vi "探头数据读取.vi"(11 "编号":string) -> ()   [LabVIEW 2016, in "斯坦道多参数.lvlib"]
panel:
  out "运行状态":u16(ring) items=["空闲", "水样测试", "标样核查"]
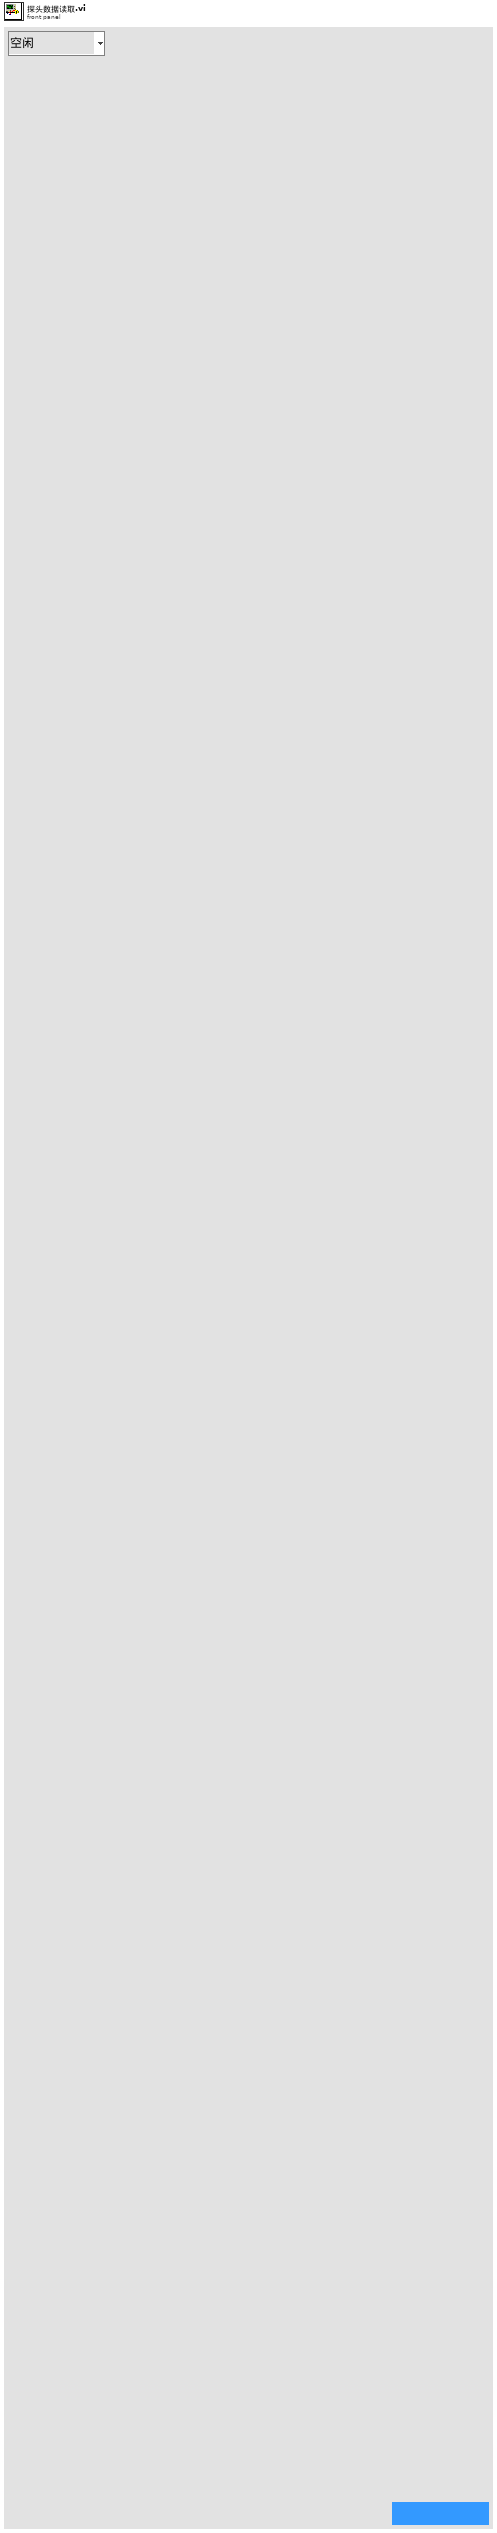
[diagram p1: front panel]
types:
  T1 = enum16{"pH", "DO", "Cond", "Turb", "ORP", "叶绿素a", "藻密度"}
  T2 = cluster{"温度测量值":sgl, "测量值":sgl, "温度偏移修正值":sgl, "信号值":sgl}
  T3 = cluster{"温度测量值":sgl, "DO%":sgl, "DOmg/L":sgl, "温度偏移修正值":sgl}
  T4 = cluster{"CH":u16, "监测值":dbl, "温度偏移修正值":sgl, "信号值":sgl}
  T5 = cluster{"pH探头选择":u16, "DO探头选择":u16, "电导率探头选择":u16, "浊度探头选择":u16, "叶绿素a探头选择":u16, "蓝绿藻探头选择":u16, "orp探头选择":u16}
  T6 = cluster{"电极状态标志":u16, "电极型号标志":u16, "酸碱度测量值":sgl, "温度测量值":sgl, "酸碱度信号值":sgl, "温度信号值":sgl, "酸碱度偏移修正值":sgl, "温度偏移修正值":sgl, "手动温度补偿值":sgl, "酸碱度电极零点":sgl, "酸碱度电极斜率":sgl, "第1点标准值记录":sgl, "第1点信号值记录":sgl, "第1点温度值记录":sgl, "第2点标准值记录":sgl, "第2点信号值记录":sgl, "第2点温度值记录":sgl, "命令滤波设定":u16, "温度模式":enum16{"ATC", "MTC"}, "生产批次":u16, "电极序号":u16, "串口地址":u16, "串口波特率":enum16{"9600", "19200", "115200"}, "串口校验位":enum16{"NONE", "ODD", "EVEN"}, "串口停止位":enum16{"1bit", "2bit"}, "第一点标准值":sgl, "第二点标准值":sgl}
  T7 = cluster{"报警码":u16, "pH数值":sgl, "0X0003_NC":sgl, "温度数据":sgl, "pH原始信号 mv":sgl, "0X0009_NC":string, "产品名称":string, "序列号":string, "硬件版本":string, "软件版本":string, "通讯地址":u16, "波特率":u16, "设备类型":u16, "0X0026_NC":string, "第一点原始数据":sgl, "第一点校准数据":sgl, "第二点原始数据":sgl, "第二点校准数据":sgl, "探头校准命令":u16, "温度校准参数":sgl, "温度校准命令":u16}
  T8 = cluster{"电极状态标志":u16, "电极型号标志":u16, "电导率测量值":sgl, "温度测量值":sgl, "电导率信号值":sgl, "温度信号值":sgl, "温度补偿系数":sgl, "电导率偏移修正值":sgl, "温度偏移修正值":sgl, "手动温度补偿值":sgl, "电导率电极零点":sgl, "电导率电极斜率":sgl, "命令滤波设定":u16, "温度模式":enum16{"ATC", "MTC"}, "生产批次":u16, "电极序号":u16, "串口地址":u16, "串口波特率":enum16{"9600", "19200", "115200"}, "串口校验位":enum16{"NONE", "ODD", "EVEN"}, "串口停止位":enum16{"1bit", "2bit"}, "第一点标准值":sgl, "第二点标准值":sgl}
  T9 = cluster{"报警码":u16, "电导率数据（uS/cm）":sgl, "0x0003 NC":sgl, "温度数据":sgl, "电导率原始信号电阻":sgl, "当前量程":u16, "温度补偿系数":sgl, "0X0009_NC":string, "产品名称":string, "序列号":string, "硬件版本":string, "软件版本":string, "通讯地址":u16, "波特率":u16, "设备类型":u16, "0X0026_NC":string, "第一点原始数据":sgl, "第一点校准数据":sgl, "0X0035_NC":sgl, "0X0037_NC":sgl, "探头校准命令":u16, "温度校准参数":sgl, "温度校准命令":u16}
  T10 = cluster{"电极状态标志":u16, "电极型号标志":u16, "溶解氧测量值":sgl, "温度测量值":sgl, "溶解氧饱和度值":sgl, "盐度补偿值":sgl, "大气压补偿值":sgl, "溶解氧偏移修正值":sgl, "温度偏移修正值":sgl, "手动温度补偿值":sgl, "溶解氧电极零点":sgl, "溶解氧电极斜率":sgl, "第1点标准值记录":sgl, "第1点信号值记录":sgl, "第1点温度值记录":sgl, "第2点标准值记录":sgl, "第2点信号值记录":sgl, "第2点温度值记录":sgl, "命令滤波设定":u16, "温度模式":enum16{"ATC", "MTC"}, "生产批次":u16, "电极序号":u16, "串口地址":u16, "串口波特率":enum16{"9600", "19200", "115200"}, "串口校验位":enum16{"NONE", "ODD", "EVEN"}, "串口停止位":enum16{"1bit", "2bit"}, "第一点标准值":sgl, "第二点标准值":sgl}
  T11 = cluster{"报警码":u16, "溶解氧数值（mg/L）":sgl, "溶解氧数据（%）":sgl, "温度数据":sgl, "溶解氧原始信号 nA":sgl, "大气压力":sgl, "盐度":sgl, "0X0009_NC":string, "产品名称":string, "序列号":string, "硬件版本":string, "软件版本":string, "通讯地址":u16, "波特率":u16, "设备类型":u16, "0X0026_NC":string, "第一点原始数据":sgl, "0X0033 NC":sgl, "第二点原始数据":sgl, "0X0037 NC":sgl, "探头校准命令":u16, "温度校准参数":sgl, "温度校准命令":u16}
  T12 = cluster{"电极状态标志":u16, "电极型号标志":u16, "浊度测量值":sgl, "温度测量值":sgl, "浊度信号值":sgl, "浊度偏移修正值":sgl, "温度偏移修正值":sgl, "手动温度补偿值":sgl, "浊度电极零点":sgl, "浊度电极斜率":sgl, "第1点标准值记录":sgl, "第1点信号值记录":sgl, "第1点温度值记录":sgl, "第2点标准值记录":sgl, "第2点信号值记录":sgl, "第2点温度值记录":sgl, "命令滤波设定":u16, "温度模式":enum16{"ATC", "MTC"}, "生产批次":u16, "电极序号":u16, "串口地址":u16, "串口波特率":enum16{"9600", "19200", "115200"}, "串口校验位":enum16{"NONE", "ODD", "EVEN"}, "串口停止位":enum16{"1bit", "2bit"}, "第一点标准值":sgl, "第二点标准值":sgl, "第三点标准值":sgl}
  T13 = cluster{"报警码":u16, "浊度数值 NTU":sgl, "温度数据":sgl, "原始光强数值":u16, "量程":u16, "平均次数":u16, "清扫模式":u16, "清扫次数":u16, "清扫间隔分钟":u16, "0X000B_NC":string, "产品名称":string, "序列号":string, "硬件版本":string, "软件版本":string, "通讯地址":u16, "波特率":u16, "设备类型":u16, "0X0026_NC":string, "校准量程":u16, "第一点原始光强":u16, "第一点校准数据":sgl, "第二点原始光强":u16, "第二点校准数据":sgl, "第三点原始光强":u16, "第三点校准数据":sgl, "探头校准命令":u16, "温度校准参数":sgl, "温度校准命令":u16}
  T14 = cluster{"电极状态标志":u16, "电极型号标志":u16, "测量值":sgl, "温度测量值":sgl, "信号值":sgl, "温度信号值":sgl, "000AH_NC":sgl, "偏移修正值":sgl, "温度偏移修正值":sgl, "手动温度补偿值":sgl, "命令滤波设定":u16, "温度模式":enum16{"ATC", "MTC"}, "生产批次":u16, "传感器序号":u16, "串口地址":u16, "串口波特率":enum16{"9600", "19200", "115200"}, "串口校验位":enum16{"NONE", "ODD", "EVEN"}, "串口停止位":enum16{"1bit", "2bit"}}
  T15 = cluster{"报警码":u16, "叶绿素a":sgl, "温度数据":sgl, "原始光强数值":u16, "量程":u16, "平均次数":u16, "清扫模式":u16, "清扫次数":u16, "清扫间隔分钟":u16, "0X000B_NC":string, "产品名称":string, "序列号":string, "硬件版本":string, "软件版本":string, "通讯地址":u16, "波特率":u16, "设备类型":u16, "0X0026_NC":string, "校准量程":u16, "第一点原始光强":u16, "第一点校准数据":sgl, "第二点原始光强":u16, "第二点校准数据":sgl, "第三点原始光强":u16, "第三点校准数据":sgl, "探头校准命令":u16, "温度校准参数":sgl, "温度校准命令":u16}
  T16 = cluster{"报警码":u16, "蓝绿藻":sgl, "温度数据":sgl, "原始光强数值":u16, "0X0006_NC":u16, "平均次数":u16, "清扫模式":u16, "清扫次数":u16, "清扫间隔分钟":u16, "0X000B_NC":string, "产品名称":string, "序列号":string, "硬件版本":string, "软件版本":string, "通讯地址":u16, "波特率":u16, "设备类型":u16, "0X0026_NC":string, "0X0030_NC":u16, "第一点原始光强":u16, "第一点校准数据":sgl, "第二点原始光强":u16, "第二点校准数据":sgl, "第三点原始光强":u16, "第三点校准数据":sgl, "探头校准命令":u16, "温度校准参数":sgl, "温度校准命令":u16}
  T17 = enum16{"pH", "DO", "Cond", "Turb", "ORP", "叶绿素a", "藻密度"}[]
  T18 = cluster{"ph":bool, "DO":bool, "Cond":bool, "Turb":bool, "叶绿素a":bool, "藻密度":bool, "ORP":bool}
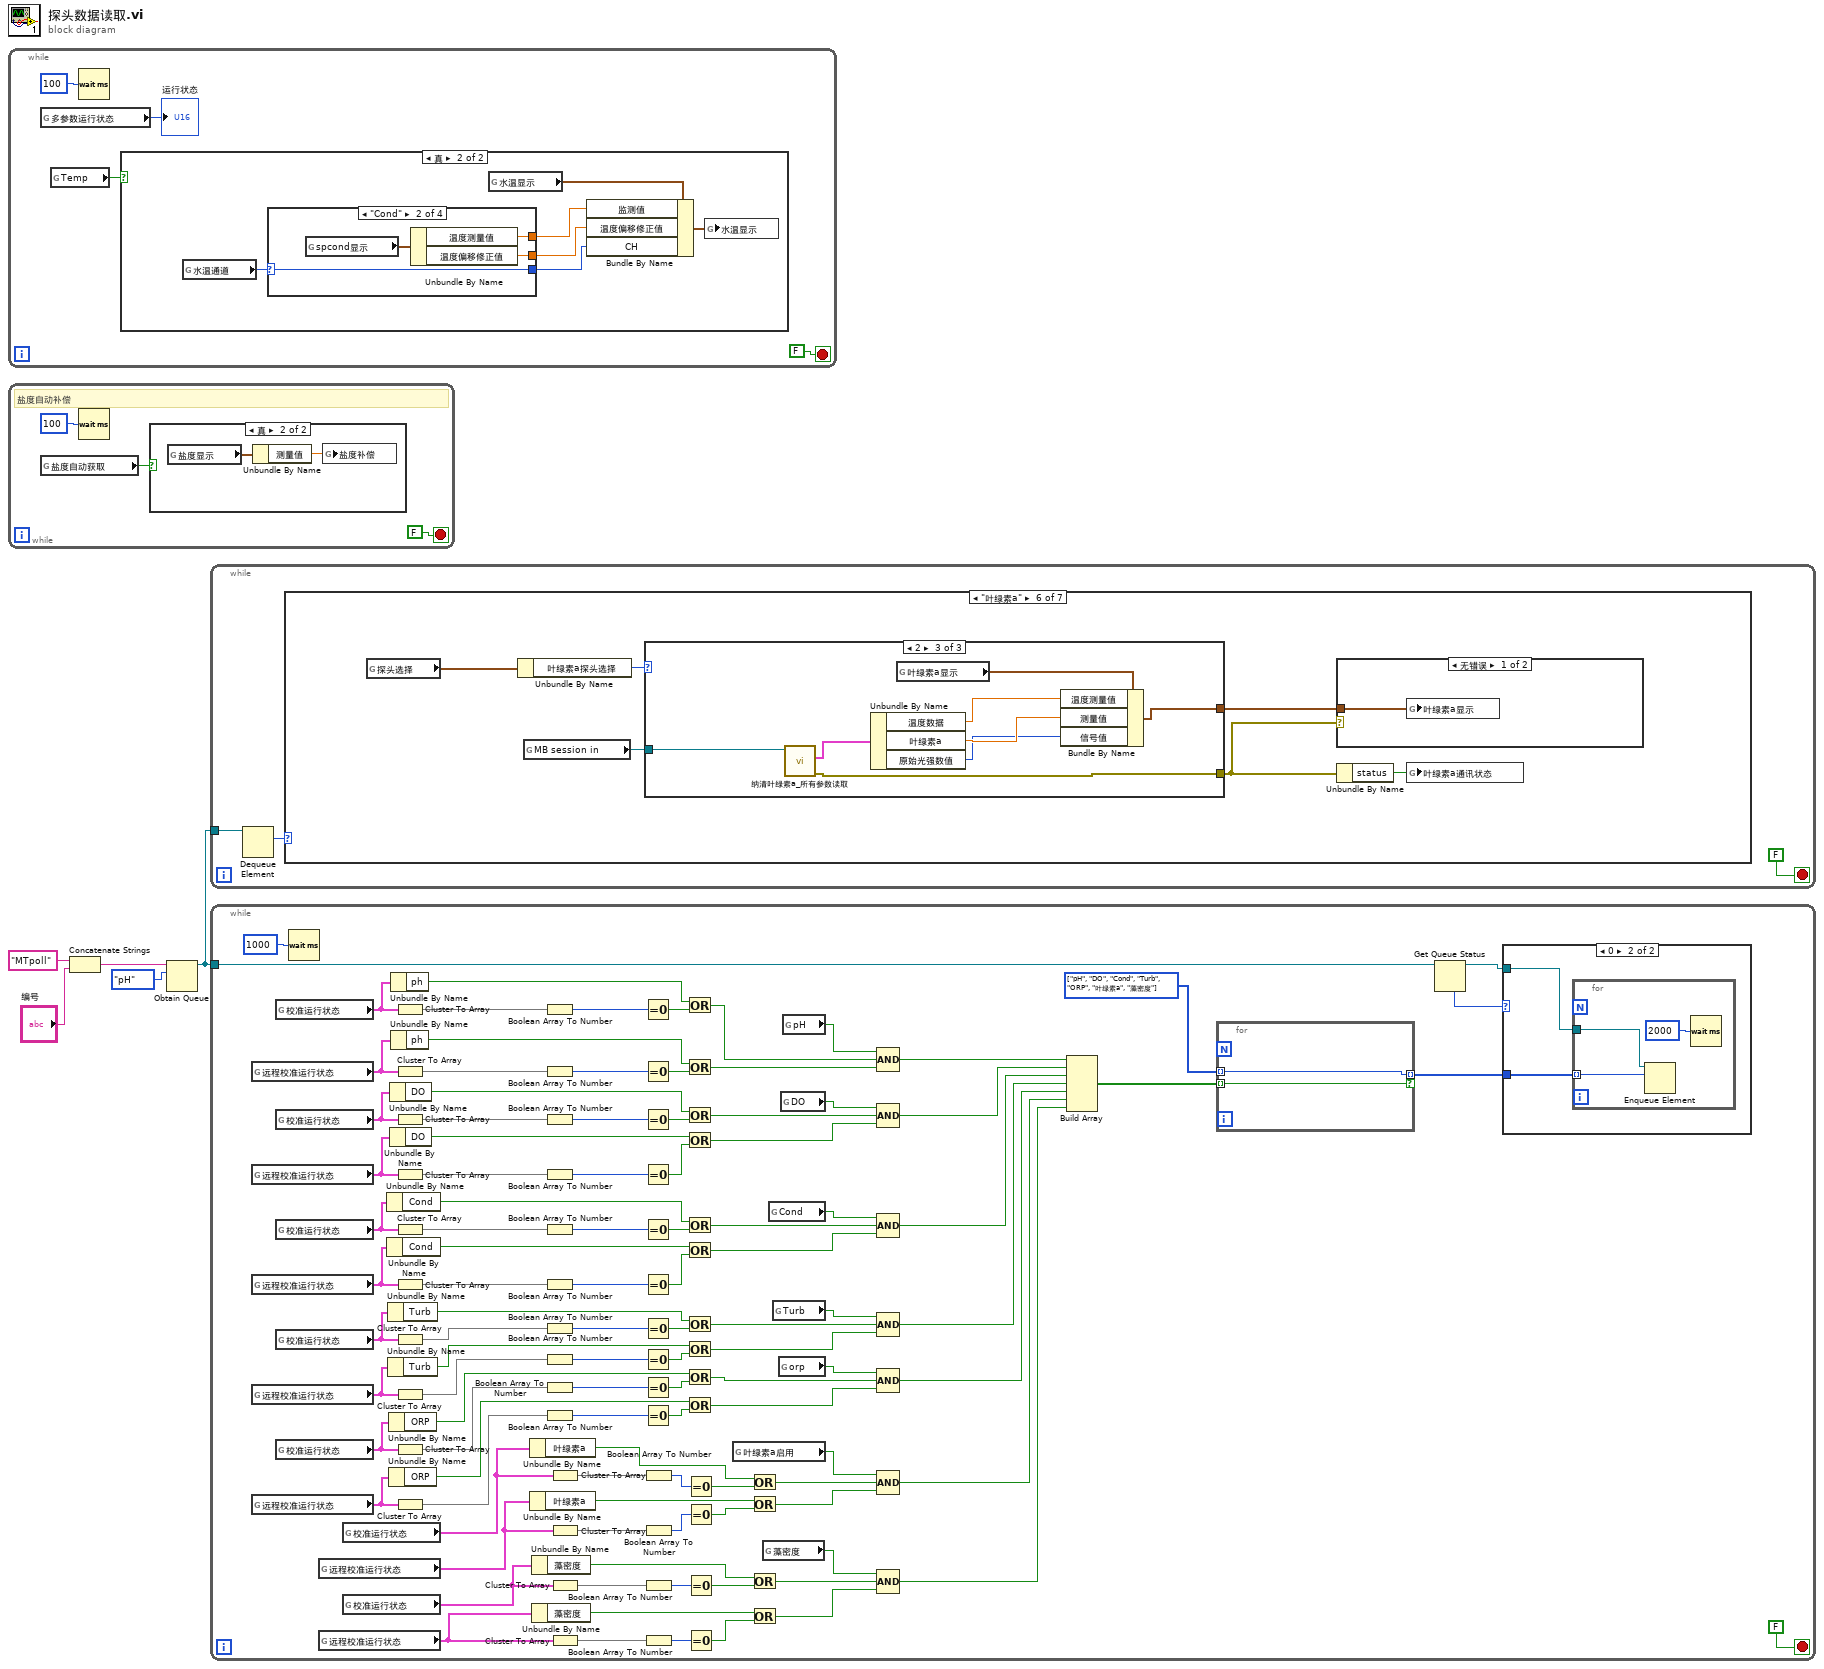
[diagram p0: block diagram]
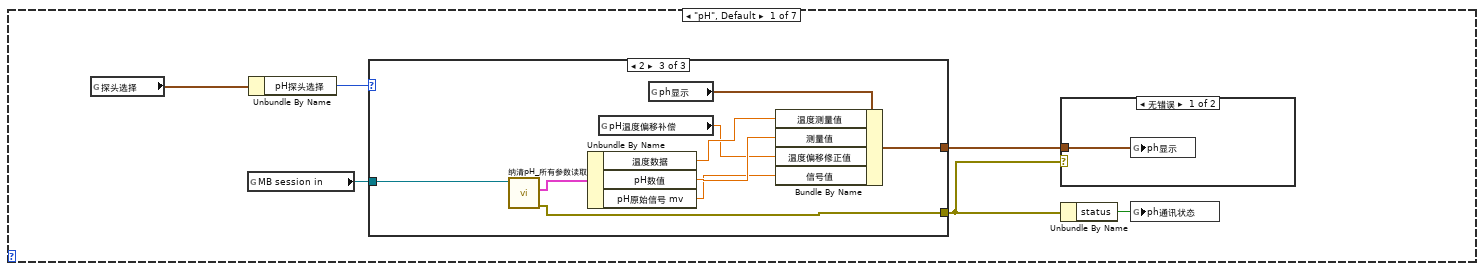
[diagram p3: hidden frame]
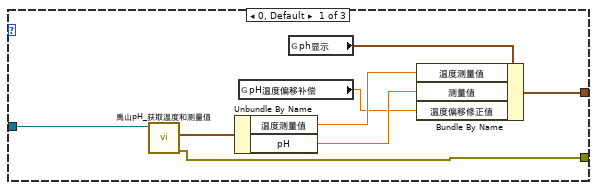
[diagram p4: hidden frame]
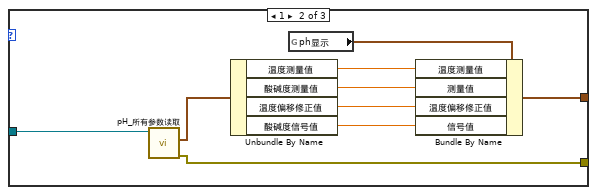
[diagram p5: hidden frame]
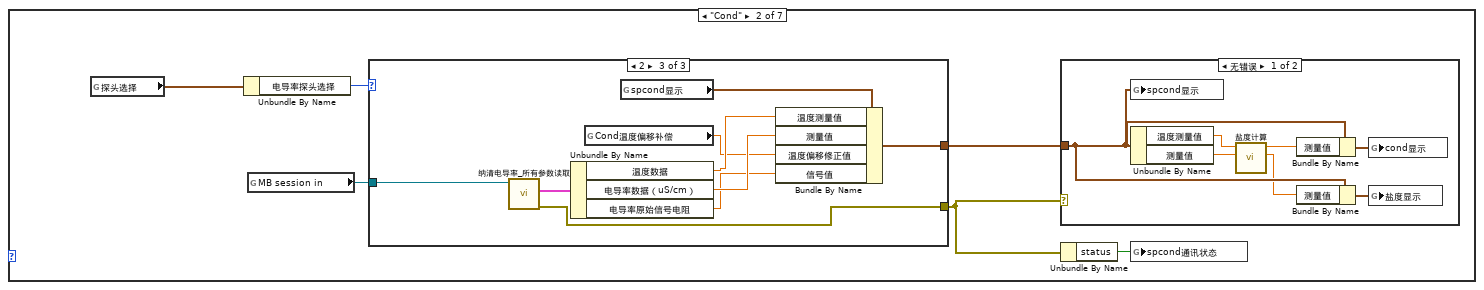
[diagram p7: hidden frame]
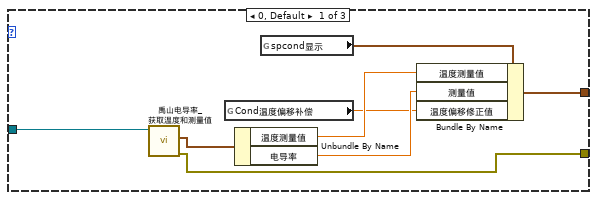
[diagram p8: hidden frame]
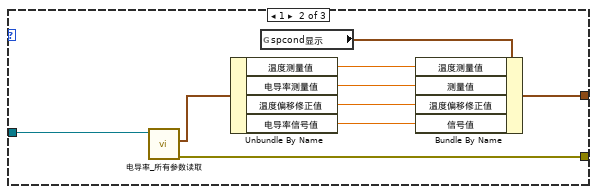
[diagram p9: hidden frame]
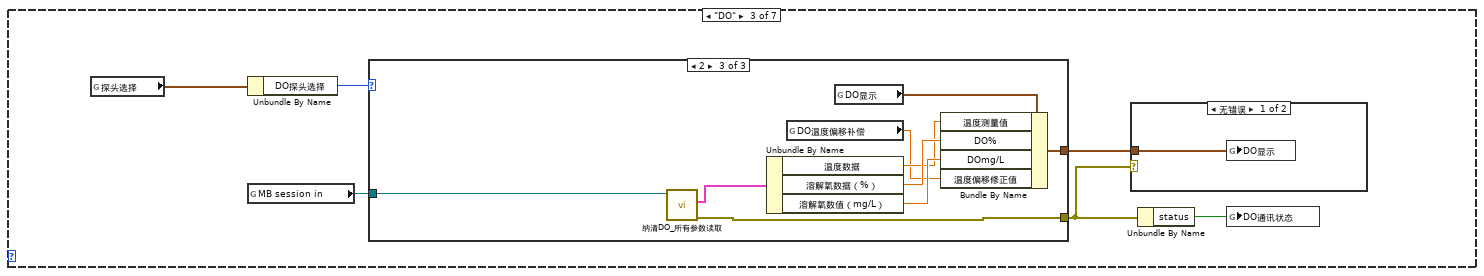
[diagram p11: hidden frame]
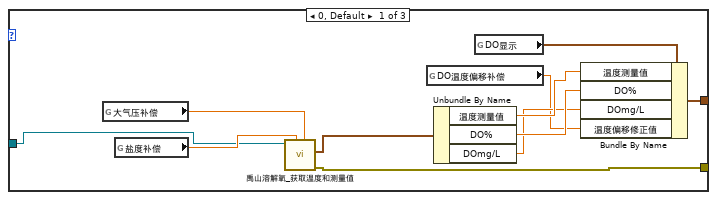
[diagram p12: hidden frame]
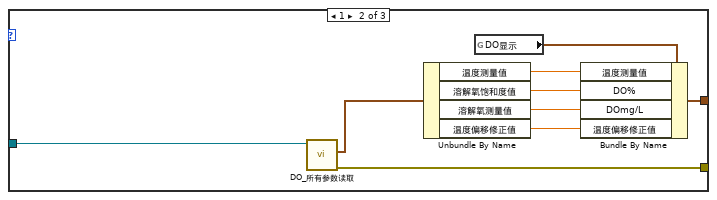
[diagram p13: hidden frame]
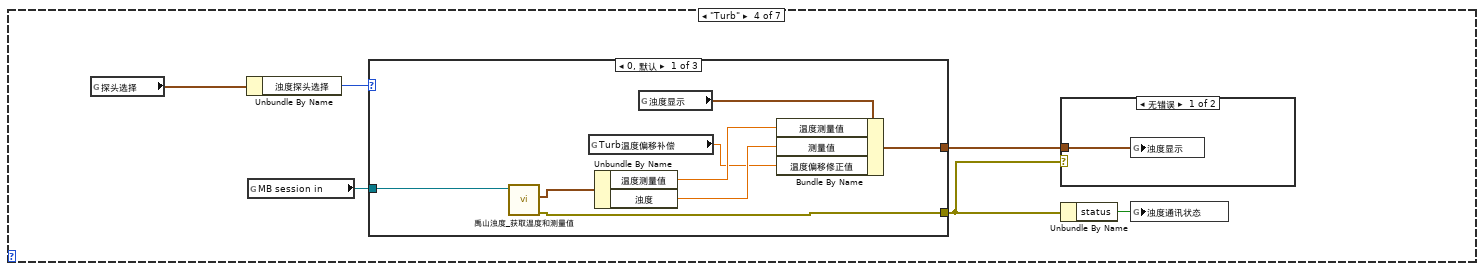
[diagram p15: hidden frame]
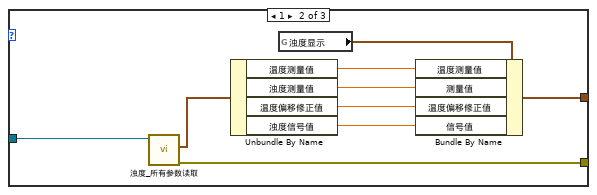
[diagram p16: hidden frame]
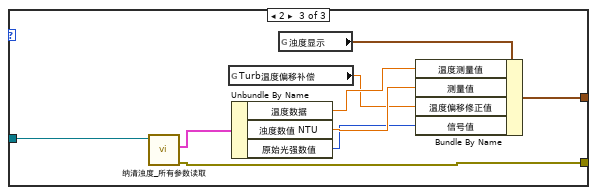
[diagram p17: hidden frame]
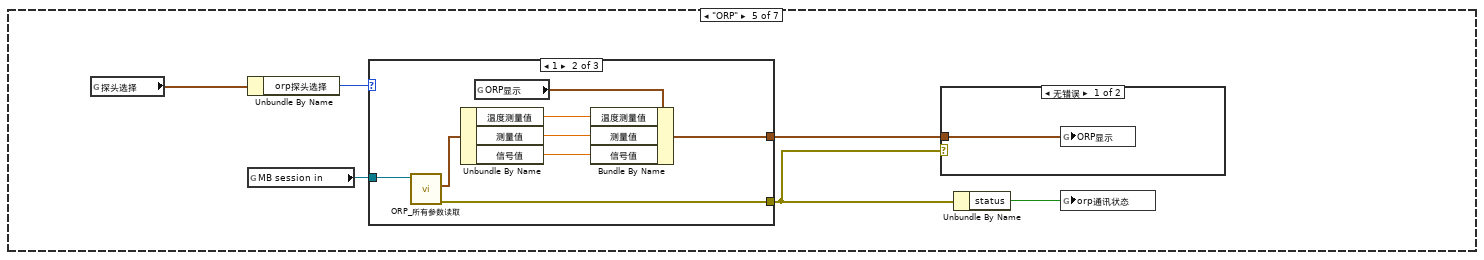
[diagram p19: hidden frame]
diagram:
  n1 = while {
    stop <- FALSE stop-if-true
    n2 = global read "多参数全局变量.vi" "多参数运行状态"() -> (→"运行状态":u16)
    n3 = global read "断电保存变量.vi" "Temp"() -> (w7:bool)
    n4 = Wait (ms)(milliseconds to wait=u32 100 ("等待时间（毫秒）")) -> ()  [unwired: 1 out]
    n5 = case shown="真" w7 {
      frame False {
      }
      frame True {
        n6 = global read "断电保存变量.vi" "水温通道"() -> (w15:enum16{"pH", "Cond", "DO", "Turb"})
        n7 = case shown="\"Cond\"" w15 {
          selector: w15 -> [w19 w23 w27 w31]
          tunnel: [w19 w23 w27 w31] -> w14
          tunnel: [w17 w20 w24 w28] -> w13
          tunnel: [w18 w21 w25 w29] -> w12
          frame "pH", Default {
            n8 = global read "多参数全局变量.vi" "ph显示"() -> (w16:T2)
            n9 = Unbundle By Name(w16) -> ("温度测量值"=w18:sgl, "温度偏移修正值"=w17:sgl)
          }
          frame "Cond" {
            n10 = global read "多参数全局变量.vi" "spcond显示"() -> (w22:T2)
            n11 = Unbundle By Name(w22) -> ("温度测量值"=w21:sgl, "温度偏移修正值"=w20:sgl)
          }
          frame "DO" {
            n12 = global read "多参数全局变量.vi" "DO显示"() -> (w26:T3)
            n13 = Unbundle By Name(w26) -> ("温度测量值"=w25:sgl, "温度偏移修正值"=w24:sgl)
          }
          frame "Turb" {
            n14 = global read "多参数全局变量.vi" "浊度显示"() -> (w30:T2)
            n15 = Unbundle By Name(w30) -> ("温度测量值"=w29:sgl, "温度偏移修正值"=w28:sgl)
          }
        }
        n16 = global read "多参数全局变量.vi" "水温显示"() -> (w10:T4)
        n17 = Bundle By Name(cluster=w10, "监测值"=w12, "温度偏移修正值"=w13, "CH"=w14) -> (w11:T4)
        n18 = global write "多参数全局变量.vi" "水温显示"(w11) -> ()
      }
    }
  }
  n19 = while {
    stop <- FALSE stop-if-true
    # "盐度自动补偿"
    n20 = global read "断电保存变量.vi" "盐度自动获取"() -> (w33:bool)
    n21 = Wait (ms)(milliseconds to wait=u32 100 ("等待时间（毫秒）")) -> ()  [unwired: 1 out]
    n22 = case shown="真" w33 {
      frame False {
      }
      frame True {
        n23 = global read "多参数全局变量.vi" "盐度显示"() -> (w36:T2)
        n24 = Unbundle By Name(w36) -> ("测量值"=w35:sgl)
        n25 = global write "断电保存变量.vi" "盐度补偿"(w35) -> ()
      }
    }
  }
  n26 = Concatenate Strings("MTpoll" ("名称（未命名）"), "编号") -> (w3:string)
  n27 = Obtain Queue(name (unnamed)=w3, element data type=T1."pH" ("枚举")) -> (queue out=w1:refnum<queue>)  [unwired: 3 in, 2 out]
  n28 = while {
    tunnel: w1 -> [w39]
    stop <- FALSE stop-if-true
    n29 = Dequeue Element(queue=w39) -> (element=w38:T1)  [unwired: 2 in, 3 out]
    n30 = case shown="\"叶绿素a\"" w38 {
      frame "pH", Default {
        n31 = global read "断电保存变量.vi" "探头选择"() -> (w45:T5)
        n32 = global read "多参数全局变量.vi" "MB session in"() -> (w43:refnum<class "MB_Master.lvclass">)
        n33 = Unbundle By Name(w45) -> ("pH探头选择"=w44:u16)
        n34 = case shown="2" w44 {
          tunnel: w43 -> [w53 w62 w69]
          tunnel: [w52 w61 w67] -> w41
          tunnel: [w50 w58 w70] -> w42
          frame 0, Default {
            n35 = call "禹山pH_获取温度和测量值.vi"("MB session in"=w53) -> ("error out"=w52:errorcluster, "输出值"=w49:cluster{"温度测量值":sgl, "ORP":sgl, "pH":sgl})  [unwired: 8 in, 1 out]
            n36 = Unbundle By Name(w49) -> ("温度测量值"=w48:sgl, "pH"=w47:sgl)
            n37 = global read "断电保存变量.vi" "pH温度偏移补偿"() -> (w46:dbl)
            n38 = global read "多参数全局变量.vi" "ph显示"() -> (w51:T2)
            n39 = Bundle By Name(cluster=w51, "温度测量值"=w48, "测量值"=w47, "温度偏移修正值"=w46) -> (w50:T2)
          }
          frame 1 {
            n40 = call "pH_所有参数读取.vi"("MB session in"=w62) -> ("error out"=w61:errorcluster, "输出值"=w60:T6)  [unwired: 8 in, 1 out]
            n41 = Unbundle By Name(w60) -> ("温度测量值"=w55:sgl, "酸碱度测量值"=w56:sgl, "温度偏移修正值"=w57:sgl, "酸碱度信号值"=w54:sgl)
            n42 = global read "多参数全局变量.vi" "ph显示"() -> (w59:T2)
            n43 = Bundle By Name(cluster=w59, "温度测量值"=w55, "测量值"=w56, "温度偏移修正值"=w57, "信号值"=w54) -> (w58:T2)
          }
          frame 2 {
            n44 = call "纳清pH_所有参数读取.vi"("MB session in"=w69) -> ("error out"=w67:errorcluster, "输出值"=w68:T7)  [unwired: 8 in, 1 out]
            n45 = Unbundle By Name(w68) -> ("温度数据"=w66:sgl, "pH数值"=w65:sgl, "pH原始信号 mv"=w63:sgl)
            n46 = global read "断电保存变量.vi" "pH温度偏移补偿"() -> (w64:dbl)
            n47 = global read "多参数全局变量.vi" "ph显示"() -> (w71:T2)
            n48 = Bundle By Name(cluster=w71, "温度测量值"=w66, "测量值"=w65, "温度偏移修正值"=w64, "信号值"=w63) -> (w70:T2)
          }
        }
        n49 = case shown="无错误" w41 {
          tunnel: w42 -> [w72 _]
          frame No Error {
            n50 = global write "多参数全局变量.vi" "ph显示"(w72) -> ()
          }
          frame Error {
          }
        }
        n51 = Unbundle By Name(w41) -> ("status"=w40:bool)
        n52 = global write "多参数全局变量.vi" "ph通讯状态"(w40) -> ()
      }
      frame "Cond" {
        n53 = global read "断电保存变量.vi" "探头选择"() -> (w78:T5)
        n54 = Unbundle By Name(w78) -> ("电导率探头选择"=w77:u16)
        n55 = global read "多参数全局变量.vi" "MB session in"() -> (w75:refnum<class "MB_Master.lvclass">)
        n56 = case shown="2" w77 {
          tunnel: w75 -> [w86 w95 w100]
          tunnel: [w80 w93 w103] -> w76
          tunnel: [w85 w92 w98] -> w74
          frame 0, Default {
            n57 = call "禹山电导率_获取温度和测量值.vi"("MB session in"=w86) -> ("error out"=w85:errorcluster, "输出值"=w83:cluster{"温度测量值":sgl, "电导率":sgl, "错误标志":u16})  [unwired: 8 in, 1 out]
            n58 = global read "断电保存变量.vi" "Cond温度偏移补偿"() -> (w79:dbl)
            n59 = Unbundle By Name(w83) -> ("温度测量值"=w82:sgl, "电导率"=w81:sgl)
            n60 = global read "多参数全局变量.vi" "spcond显示"() -> (w84:T2)
            n61 = Bundle By Name(cluster=w84, "温度测量值"=w82, "测量值"=w81, "温度偏移修正值"=w79) -> (w80:T2)
          }
          frame 1 {
            n62 = call "电导率_所有参数读取.vi"("MB session in"=w95) -> ("error out"=w92:errorcluster, "输出值"=w91:T8)  [unwired: 8 in, 1 out]
            n63 = Unbundle By Name(w91) -> ("温度测量值"=w90:sgl, "电导率测量值"=w89:sgl, "温度偏移修正值"=w88:sgl, "电导率信号值"=w87:sgl)
            n64 = global read "多参数全局变量.vi" "spcond显示"() -> (w94:T2)
            n65 = Bundle By Name(cluster=w94, "温度测量值"=w90, "测量值"=w89, "温度偏移修正值"=w88, "信号值"=w87) -> (w93:T2)
          }
          frame 2 {
            n66 = call "纳清电导率_所有参数读取.vi"("MB session in"=w100) -> ("error out"=w98:errorcluster, "输出值"=w99:T9)  [unwired: 8 in, 1 out]
            n67 = Unbundle By Name(w99) -> ("温度数据"=w102:sgl, "电导率数据（uS/cm）"=w101:sgl, "电导率原始信号电阻"=w96:sgl)
            n68 = global read "断电保存变量.vi" "Cond温度偏移补偿"() -> (w97:dbl)
            n69 = global read "多参数全局变量.vi" "spcond显示"() -> (w104:T2)
            n70 = Bundle By Name(cluster=w104, "温度测量值"=w102, "测量值"=w101, "温度偏移修正值"=w97, "信号值"=w96) -> (w103:T2)
          }
        }
        n71 = case shown="无错误" w74 {
          tunnel: w76 -> [w106 _]
          frame No Error {
            n72 = global write "多参数全局变量.vi" "spcond显示"(w106) -> ()
            n73 = Unbundle By Name(w106) -> ("温度测量值"=w111:sgl, "测量值"=w110:sgl)
            n74 = call "盐度计算.vi"("spCond"=w110, "Temp"=w111) -> ("saltresult"=w105:dbl, "cond"=w109:dbl)  [unwired: 8 in]
            n75 = Bundle By Name(cluster=w106, "测量值"=w109) -> (w108:T2)
            n76 = Bundle By Name(cluster=w106, "测量值"=w105) -> (w107:T2)
            n77 = global write "多参数全局变量.vi" "cond显示"(w108) -> ()
            n78 = global write "多参数全局变量.vi" "盐度显示"(w107) -> ()
          }
          frame Error {
          }
        }
        n79 = Unbundle By Name(w74) -> ("status"=w73:bool)
        n80 = global write "多参数全局变量.vi" "spcond通讯状态"(w73) -> ()
      }
      frame "DO" {
        n81 = global read "断电保存变量.vi" "探头选择"() -> (w117:T5)
        n82 = Unbundle By Name(w117) -> ("DO探头选择"=w116:u16)
        n83 = global read "多参数全局变量.vi" "MB session in"() -> (w114:refnum<class "MB_Master.lvclass">)
        n84 = case shown="2" w116 {
          tunnel: w114 -> [w126 w137 w141]
          tunnel: [w124 w135 w145] -> w115
          tunnel: [w120 w130 w139] -> w113
          frame 0, Default {
            n85 = global read "断电保存变量.vi" "大气压补偿"() -> (w127:dbl)
            n86 = global read "断电保存变量.vi" "盐度补偿"() -> (w128:dbl)
            n87 = call "禹山溶解氧_获取温度和测量值.vi"("大气压补偿"=w127, "盐度补偿"=w128, "MB session in"=w126) -> ("error out"=w120:errorcluster, "输出值"=w118:cluster{"温度测量值":sgl, "DO%":sgl, "DOmg/L":sgl})  [unwired: 6 in, 1 out]
            n88 = global read "断电保存变量.vi" "DO温度偏移补偿"() -> (w119:dbl)
            n89 = Unbundle By Name(w118) -> ("温度测量值"=w123:sgl, "DO%"=w122:sgl, "DOmg/L"=w121:sgl)
            n90 = global read "多参数全局变量.vi" "DO显示"() -> (w125:T3)
            n91 = Bundle By Name(cluster=w125, "温度测量值"=w123, "DO%"=w122, "DOmg/L"=w121, "温度偏移修正值"=w119) -> (w124:T3)
          }
          frame 1 {
            n92 = call "DO_所有参数读取.vi"("MB session in"=w137) -> ("error out"=w130:errorcluster, "输出值"=w134:T10)  [unwired: 8 in, 1 out]
            n93 = Unbundle By Name(w134) -> ("温度测量值"=w131:sgl, "溶解氧饱和度值"=w132:sgl, "溶解氧测量值"=w133:sgl, "温度偏移修正值"=w129:sgl)
            n94 = global read "多参数全局变量.vi" "DO显示"() -> (w136:T3)
            n95 = Bundle By Name(cluster=w136, "温度测量值"=w131, "DO%"=w132, "DOmg/L"=w133, "温度偏移修正值"=w129) -> (w135:T3)
          }
          frame 2 {
            n96 = call "纳清DO_所有参数读取.vi"("MB session in"=w141) -> ("error out"=w139:errorcluster, "输出值"=w140:T11)  [unwired: 8 in, 1 out]
            n97 = Unbundle By Name(w140) -> ("温度数据"=w142:sgl, "溶解氧数据（%）"=w143:sgl, "溶解氧数值（mg/L）"=w144:sgl)
            n98 = global read "断电保存变量.vi" "DO温度偏移补偿"() -> (w138:dbl)
            n99 = global read "多参数全局变量.vi" "DO显示"() -> (w146:T3)
            n100 = Bundle By Name(cluster=w146, "温度测量值"=w142, "DO%"=w143, "DOmg/L"=w144, "温度偏移修正值"=w138) -> (w145:T3)
          }
        }
        n101 = case shown="无错误" w113 {
          tunnel: w115 -> [w147 _]
          frame No Error {
            n102 = global write "多参数全局变量.vi" "DO显示"(w147) -> ()
          }
          frame Error {
          }
        }
        n103 = Unbundle By Name(w113) -> ("status"=w112:bool)
        n104 = global write "多参数全局变量.vi" "DO通讯状态"(w112) -> ()
      }
      frame "Turb" {
        n105 = global read "断电保存变量.vi" "探头选择"() -> (w153:T5)
        n106 = Unbundle By Name(w153) -> ("浊度探头选择"=w152:u16)
        n107 = global read "多参数全局变量.vi" "MB session in"() -> (w150:refnum<class "MB_Master.lvclass">)
        n108 = case shown="0, 默认" w152 {
          tunnel: w150 -> [w161 w170 w175]
          tunnel: [w159 w165 w176] -> w151
          tunnel: [w158 w164 w174] -> w149
          frame 0, Default {
            n109 = call "禹山浊度_获取温度和测量值.vi"("MB session in"=w161) -> ("error out"=w158:errorcluster, "输出值"=w157:cluster{"温度测量值":sgl, "浊度":sgl})  [unwired: 8 in, 1 out]
            n110 = global read "断电保存变量.vi" "Turb温度偏移补偿"() -> (w154:dbl)
            n111 = Unbundle By Name(w157) -> ("温度测量值"=w156:sgl, "浊度"=w155:sgl)
            n112 = global read "多参数全局变量.vi" "浊度显示"() -> (w160:T2)
            n113 = Bundle By Name(cluster=w160, "温度测量值"=w156, "测量值"=w155, "温度偏移修正值"=w154) -> (w159:T2)
          }
          frame 1 {
            n114 = call "浊度_所有参数读取.vi"("MB session in"=w170) -> ("error out"=w164:errorcluster, "输出值"=w169:T12)  [unwired: 8 in, 1 out]
            n115 = Unbundle By Name(w169) -> ("温度测量值"=w167:sgl, "浊度测量值"=w166:sgl, "温度偏移修正值"=w163:sgl, "浊度信号值"=w162:sgl)
            n116 = global read "多参数全局变量.vi" "浊度显示"() -> (w168:T2)
            n117 = Bundle By Name(cluster=w168, "温度测量值"=w167, "测量值"=w166, "温度偏移修正值"=w163, "信号值"=w162) -> (w165:T2)
          }
          frame 2 {
            n118 = call "纳清浊度_所有参数读取.vi"("MB session in"=w175) -> ("error out"=w174:errorcluster, "输出值"=w173:T13)  [unwired: 8 in, 1 out]
            n119 = global read "断电保存变量.vi" "Turb温度偏移补偿"() -> (w172:dbl)
            n120 = Unbundle By Name(w173) -> ("温度数据"=w178:sgl, "浊度数值 NTU"=w177:sgl, "原始光强数值"=w171:u16)
            n121 = global read "多参数全局变量.vi" "浊度显示"() -> (w179:T2)
            n122 = Bundle By Name(cluster=w179, "温度测量值"=w178, "测量值"=w177, "温度偏移修正值"=w172, "信号值"=w171) -> (w176:T2)
          }
        }
        n123 = case shown="无错误" w149 {
          tunnel: w151 -> [w180 _]
          frame No Error {
            n124 = global write "多参数全局变量.vi" "浊度显示"(w180) -> ()
          }
          frame Error {
          }
        }
        n125 = Unbundle By Name(w149) -> ("status"=w148:bool)
        n126 = global write "多参数全局变量.vi" "浊度通讯状态"(w148) -> ()
      }
      frame "ORP" {
        n127 = global read "断电保存变量.vi" "探头选择"() -> (w185:T5)
        n128 = Unbundle By Name(w185) -> ("orp探头选择"=w184:u16)
        n129 = global read "多参数全局变量.vi" "MB session in"() -> (w183:refnum<class "MB_Master.lvclass">)
        n130 = case shown="1" w184 {
          tunnel: [_ w189 _] -> w182
          tunnel: w183 -> [_ w194 _]
          tunnel: [_ w187 _] -> w186
          frame 0, Default {
          }
          frame 1 {
            n131 = call "ORP_所有参数读取.vi"("MB session in"=w194) -> ("error out"=w189:errorcluster, "输出值"=w191:T14)  [unwired: 8 in, 1 out]
            n132 = Unbundle By Name(w191) -> ("温度测量值"=w192:sgl, "测量值"=w193:sgl, "信号值"=w188:sgl)
            n133 = global read "多参数全局变量.vi" "ORP显示"() -> (w190:T2)
            n134 = Bundle By Name(cluster=w190, "温度测量值"=w192, "测量值"=w193, "信号值"=w188) -> (w187:T2)
          }
          frame 2 {
          }
        }
        n135 = case shown="无错误" w182 {
          tunnel: w186 -> [w195 _]
          frame No Error {
            n136 = global write "多参数全局变量.vi" "ORP显示"(w195) -> ()
          }
          frame Error {
          }
        }
        n137 = Unbundle By Name(w182) -> ("status"=w181:bool)
        n138 = global write "多参数全局变量.vi" "orp通讯状态"(w181) -> ()
      }
      frame "叶绿素a" {
        n139 = global read "断电保存变量.vi" "探头选择"() -> (w200:T5)
        n140 = Unbundle By Name(w200) -> ("叶绿素a探头选择"=w199:u16)
        n141 = global read "多参数全局变量.vi" "MB session in"() -> (w198:refnum<class "MB_Master.lvclass">)
        n142 = case shown="2" w199 {
          tunnel: [w208 _ w214] -> w197
          tunnel: w198 -> [w207 _ w216]
          tunnel: [w205 _ w213] -> w201
          frame 0, Default {
            n143 = call "叶绿素a_获取温度和叶绿素值.vi"("MB session in"=w207) -> ("error out"=w208:errorcluster, "输出值"=w204:cluster{"温度测量值":sgl, "叶绿素测量值":sgl, "错误标志":u16})  [unwired: 8 in, 1 out]
            n144 = Unbundle By Name(w204) -> ("温度测量值"=w202:sgl, "叶绿素测量值"=w203:sgl)
            n145 = global read "多参数全局变量.vi" "叶绿素a显示"() -> (w206:T2)
            n146 = Bundle By Name(cluster=w206, "温度测量值"=w202, "测量值"=w203) -> (w205:T2)
          }
          frame 1 {
          }
          frame 2 {
            n147 = call "纳清叶绿素a_所有参数读取.vi"("MB session in"=w216) -> ("error out"=w214:errorcluster, "输出值"=w212:T15)  [unwired: 8 in, 1 out]
            n148 = Unbundle By Name(w212) -> ("温度数据"=w210:sgl, "叶绿素a"=w211:sgl, "原始光强数值"=w209:u16)
            n149 = global read "多参数全局变量.vi" "叶绿素a显示"() -> (w215:T2)
            n150 = Bundle By Name(cluster=w215, "温度测量值"=w210, "测量值"=w211, "信号值"=w209) -> (w213:T2)
          }
        }
        n151 = case shown="无错误" w197 {
          tunnel: w201 -> [w217 _]
          frame No Error {
            n152 = global write "多参数全局变量.vi" "叶绿素a显示"(w217) -> ()
          }
          frame Error {
          }
        }
        n153 = Unbundle By Name(w197) -> ("status"=w196:bool)
        n154 = global write "多参数全局变量.vi" "叶绿素a通讯状态"(w196) -> ()
      }
      frame "藻密度" {
        n155 = global read "断电保存变量.vi" "探头选择"() -> (w222:T5)
        n156 = Unbundle By Name(w222) -> ("蓝绿藻探头选择"=w221:u16)
        n157 = global read "多参数全局变量.vi" "MB session in"() -> (w220:refnum<class "MB_Master.lvclass">)
        n158 = case shown="2" w221 {
          tunnel: [_ _ w229] -> w219
          tunnel: w220 -> [_ _ w231]
          tunnel: [_ _ w228] -> w223
          frame 0, Default {
          }
          frame 1 {
          }
          frame 2 {
            n159 = call "纳清蓝绿藻_所有参数读取.vi"("MB session in"=w231) -> ("error out"=w229:errorcluster, "输出值"=w227:T16)  [unwired: 8 in, 1 out]
            n160 = Unbundle By Name(w227) -> ("温度数据"=w226:sgl, "蓝绿藻"=w225:sgl, "原始光强数值"=w224:u16)
            n161 = global read "多参数全局变量.vi" "藻密度显示"() -> (w230:T2)
            n162 = Bundle By Name(cluster=w230, "温度测量值"=w226, "测量值"=w225, "信号值"=w224) -> (w228:T2)
          }
        }
        n163 = case shown="无错误" w219 {
          tunnel: w223 -> [w232 _]
          frame No Error {
            n164 = global write "多参数全局变量.vi" "藻密度显示"(w232) -> ()
          }
          frame Error {
          }
        }
        n165 = Unbundle By Name(w219) -> ("status"=w218:bool)
        n166 = global write "多参数全局变量.vi" "藻密度通讯状态"(w218) -> ()
      }
    }
  }
  n167 = while {
    tunnel: w1 -> [w338]
    stop <- FALSE stop-if-true
    w237 = T17 [enum."pH", enum."DO", enum."Cond", enum."Turb", enum."ORP", enum."叶绿素a", enum."藻密度"] items=["pH", "DO", "Cond", "Turb", "ORP", "叶绿素a", "藻密度"]
    n168 = global read "多参数全局变量.vi" "远程校准运行状态"() -> (w335:T18)
    n169 = global read "多参数全局变量.vi" "远程校准运行状态"() -> (w309:T18)
    n170 = global read "多参数全局变量.vi" "远程校准运行状态"() -> (w312:T18)
    n171 = global read "多参数全局变量.vi" "远程校准运行状态"() -> (w296:T18)
    n172 = global read "多参数全局变量.vi" "远程校准运行状态"() -> (w283:T18)
    n173 = global read "多参数全局变量.vi" "校准运行状态"() -> (w324:T18)
    n174 = global read "多参数全局变量.vi" "校准运行状态"() -> (w298:T18)
    n175 = global read "多参数全局变量.vi" "校准运行状态"() -> (w323:T18)
    n176 = global read "多参数全局变量.vi" "校准运行状态"() -> (w285:T18)
    n177 = global read "多参数全局变量.vi" "校准运行状态"() -> (w272:T18)
    n178 = Wait (ms)(milliseconds to wait=u32 1000 ("等待时间（毫秒）")) -> ()  [unwired: 1 out]
    n179 = global read "多参数全局变量.vi" "远程校准运行状态"() -> (w260:T18)
    n180 = global read "多参数全局变量.vi" "远程校准运行状态"() -> (w257:T18)
    n181 = global read "多参数全局变量.vi" "校准运行状态"() -> (w271:T18)
    n182 = global read "多参数全局变量.vi" "校准运行状态"() -> (w246:T18)
    n183 = Unbundle By Name(w323) -> ("Cond"=w321:bool)
    n184 = Unbundle By Name(w312) -> ("Cond"=w313:bool)
    n185 = Unbundle By Name(w285) -> ("Turb"=w287:bool)
    n186 = Unbundle By Name(w296) -> ("Turb"=w295:bool)
    n187 = Unbundle By Name(w272) -> ("ORP"=w274:bool)
    n188 = Unbundle By Name(w283) -> ("ORP"=w282:bool)
    n189 = Unbundle By Name(w298) -> ("DO"=w300:bool)
    n190 = Unbundle By Name(w309) -> ("DO"=w308:bool)
    n191 = Unbundle By Name(w324) -> ("ph"=w326:bool)
    n192 = Unbundle By Name(w335) -> ("ph"=w334:bool)
    n193 = Cluster To Array(cluster=w324) -> (array=w329:bool[])
    n194 = Cluster To Array(cluster=w335) -> (array=w331:bool[])
    n195 = Cluster To Array(cluster=w298) -> (array=w303:bool[])
    n196 = Cluster To Array(cluster=w309) -> (array=w305:bool[])
    n197 = Cluster To Array(cluster=w323) -> (array=w318:bool[])
    n198 = Cluster To Array(cluster=w312) -> (array=w316:bool[])
    n199 = Cluster To Array(cluster=w285) -> (array=w290:bool[])
    n200 = Cluster To Array(cluster=w296) -> (array=w292:bool[])
    n201 = Cluster To Array(cluster=w272) -> (array=w277:bool[])
    n202 = Cluster To Array(cluster=w283) -> (array=w279:bool[])
    n203 = Unbundle By Name(w271) -> ("叶绿素a"=w269:bool)
    n204 = Unbundle By Name(w260) -> ("叶绿素a"=w261:bool)
    n205 = Unbundle By Name(w246) -> ("藻密度"=w248:bool)
    n206 = Unbundle By Name(w257) -> ("藻密度"=w256:bool)
    n207 = Boolean Array To Number(Boolean array=w329) -> (number=w328:u32)
    n208 = Boolean Array To Number(Boolean array=w331) -> (number=w332:u32)
    n209 = Boolean Array To Number(Boolean array=w303) -> (number=w302:u32)
    n210 = Boolean Array To Number(Boolean array=w305) -> (number=w306:u32)
    n211 = Boolean Array To Number(Boolean array=w318) -> (number=w319:u32)
    n212 = Boolean Array To Number(Boolean array=w316) -> (number=w315:u32)
    n213 = Boolean Array To Number(Boolean array=w290) -> (number=w289:u32)
    n214 = Boolean Array To Number(Boolean array=w292) -> (number=w293:u32)
    n215 = Boolean Array To Number(Boolean array=w277) -> (number=w276:u32)
    n216 = Boolean Array To Number(Boolean array=w279) -> (number=w280:u32)
    n217 = Cluster To Array(cluster=w271) -> (array=w266:bool[])
    n218 = Cluster To Array(cluster=w260) -> (array=w264:bool[])
    n219 = Cluster To Array(cluster=w246) -> (array=w251:bool[])
    n220 = Cluster To Array(cluster=w257) -> (array=w253:bool[])
    n221 = Equal To 0?(x=w328) -> (x = 0?=w327:bool)
    n222 = Equal To 0?(x=w332) -> (x = 0?=w333:bool)
    n223 = Equal To 0?(x=w302) -> (x = 0?=w301:bool)
    n224 = Equal To 0?(x=w306) -> (x = 0?=w307:bool)
    n225 = Equal To 0?(x=w319) -> (x = 0?=w320:bool)
    n226 = Equal To 0?(x=w315) -> (x = 0?=w314:bool)
    n227 = Equal To 0?(x=w289) -> (x = 0?=w288:bool)
    n228 = Equal To 0?(x=w293) -> (x = 0?=w294:bool)
    n229 = Equal To 0?(x=w276) -> (x = 0?=w275:bool)
    n230 = Equal To 0?(x=w280) -> (x = 0?=w281:bool)
    n231 = Boolean Array To Number(Boolean array=w266) -> (number=w267:u32)
    n232 = Boolean Array To Number(Boolean array=w264) -> (number=w263:u32)
    n233 = Boolean Array To Number(Boolean array=w251) -> (number=w250:u32)
    n234 = Boolean Array To Number(Boolean array=w253) -> (number=w254:u32)
    n235 = Or(x=w326, y=w327) -> (x .or. y?=w325:bool)
    n236 = Or(x=w334, y=w333) -> (x .or. y?=w336:bool)
    n237 = Or(x=w300, y=w301) -> (x .or. y?=w299:bool)
    n238 = Or(x=w308, y=w307) -> (x .or. y?=w310:bool)
    n239 = Or(x=w321, y=w320) -> (x .or. y?=w322:bool)
    n240 = Or(x=w313, y=w314) -> (x .or. y?=w311:bool)
    n241 = Or(x=w287, y=w288) -> (x .or. y?=w286:bool)
    n242 = Or(x=w295, y=w294) -> (x .or. y?=w297:bool)
    n243 = Or(x=w274, y=w275) -> (x .or. y?=w273:bool)
    n244 = Or(x=w282, y=w281) -> (x .or. y?=w284:bool)
    n245 = Equal To 0?(x=w267) -> (x = 0?=w268:bool)
    n246 = Equal To 0?(x=w263) -> (x = 0?=w262:bool)
    n247 = Equal To 0?(x=w250) -> (x = 0?=w249:bool)
    n248 = Equal To 0?(x=w254) -> (x = 0?=w255:bool)
    n249 = global read "断电保存变量.vi" "叶绿素a启用"() -> (w265:bool)
    n250 = Or(x=w269, y=w268) -> (x .or. y?=w270:bool)
    n251 = Or(x=w261, y=w262) -> (x .or. y?=w259:bool)
    n252 = Or(x=w248, y=w249) -> (x .or. y?=w247:bool)
    n253 = Or(x=w256, y=w255) -> (x .or. y?=w258:bool)
    n254 = global read "断电保存变量.vi" "藻密度"() -> (w252:bool)
    n255 = global read "断电保存变量.vi" "Cond"() -> (w317:bool)
    n256 = global read "断电保存变量.vi" "Turb"() -> (w291:bool)
    n257 = global read "断电保存变量.vi" "orp"() -> (w278:bool)
    n258 = global read "断电保存变量.vi" "DO"() -> (w304:bool)
    n259 = global read "断电保存变量.vi" "pH"() -> (w330:bool)
    n260 = Compound Arithmetic op=AND ("复合运算")(w330, w325, w336) -> (w245:bool)
    n261 = Compound Arithmetic op=AND ("复合运算")(w304, w299, w310) -> (w244:bool)
    n262 = Compound Arithmetic op=AND ("复合运算")(w317, w322, w311) -> (w243:bool)
    n263 = Compound Arithmetic op=AND ("复合运算")(w291, w286, w297) -> (w242:bool)
    n264 = Compound Arithmetic op=AND ("复合运算")(w278, w273, w284) -> (w241:bool)
    n265 = Compound Arithmetic op=AND ("复合运算")(w265, w270, w259) -> (w240:bool)
    n266 = Compound Arithmetic op=AND ("复合运算")(w252, w247, w258) -> (w239:bool)
    n267 = Build Array(w245, w244, w243, w242, w241, w240, w239) -> (w238:bool[])
    n268 = for {
      tunnel: w238 -> [w344] mode=indexing
      tunnel: w237 -> [w345] mode=indexing
      tunnel: [w345] -> w236 mode=indexing if=w344
    }
    n269 = Get Queue Status(queue=w338) -> (queue out=w234:refnum<queue>, # elements in queue=w233:i32)  [unwired: 2 in, 6 out]
    n270 = case shown="0" w233 {
      tunnel: w236 -> [_ w340]
      tunnel: w234 -> [_ w339]
      frame Default {
      }
      frame 0 {
        n271 = for {
          tunnel: w339 -> [w343]
          tunnel: w340 -> [w342] mode=indexing
          n272 = Enqueue Element(queue=w343, element=w342) -> ()  [unwired: 2 in, 3 out]
          n273 = Wait (ms)(milliseconds to wait=u32 2000 ("等待时间（毫秒）")) -> ()  [unwired: 1 out]
        }
      }
    }
  }
